vi "MT EbN0 Calculation(ASK).vi"(0 "Recieved waveform":T3={"t0"=0.0, "dt"=1.0, "Y"=[]} {"Y" format="%.3f"; "dt" format="%^.2e"; "t0" format="%.4f"}, 1 "pulse shaping filter coefficients":dbl[](array[numeric]) format="%.2f", 5 "ASK system parameters":T1={"samples per symbol (16)"=16, "symbol map"=[]} {"symbol map" format="%.3f"}, 7 "synchronization parameters":T2 {"sync sequence" format="%.2f"}, 9 "matched filter coefficients":dbl[](array[numeric]) format="%.2f", 11 "error in (no error)":errorcluster, 12 "reset? (T)":bool=TRUE) -> (4 "Eb/N0":dbl, 6 "Eb/N0(dB)":dbl, 15 "error out":errorcluster)   [LabVIEW 2020, in "niDMT.lvlib"]
uses:
  <vilib>/addons/Modulation/niDMT.lvlib
  <vilib>/addons/Modulation/Analog/controls/Complex Data Waveform.ctl
  <vilib>/Analysis/2dsp.llb/1D Convolution (DBL).vi
  <vilib>/Analysis/NI_AALPro.lvlib
  <vilib>/addons/Modulation/niAMT.lvlib
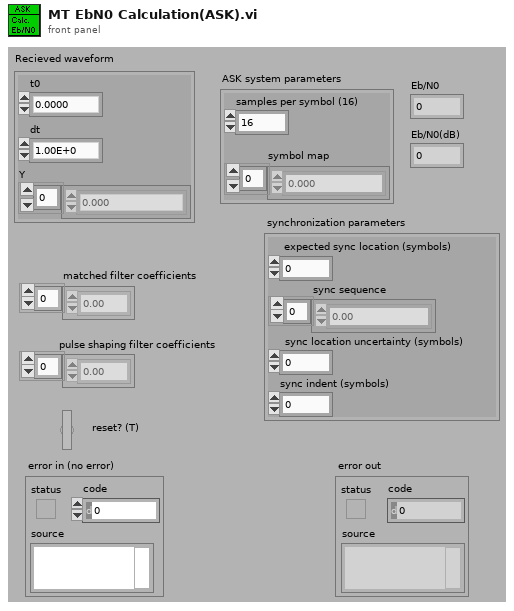
[diagram p1: front panel]
types:
  T1 = cluster{"samples per symbol (16)":i32, "symbol map":cdb[]}
  T2 = cluster{"expected sync location (symbols)":i32, "sync sequence":cdb[], "sync location uncertainty (symbols)":i32, "sync indent (symbols)":i32}
  T3 = typedef "niAMT.lvlib/Complex Data Waveform.ctl" = cluster{"t0":dbl, "dt":dbl, "Y":cdb[]}
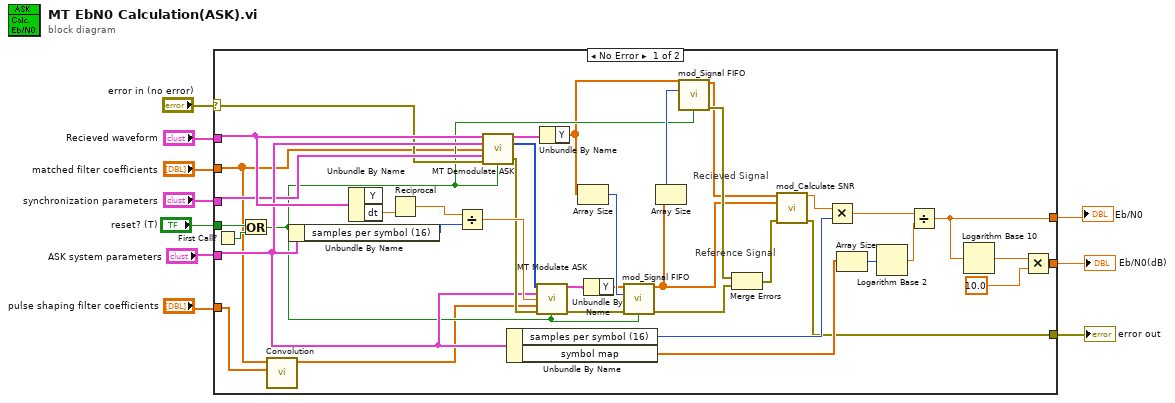
[diagram p0: block diagram]
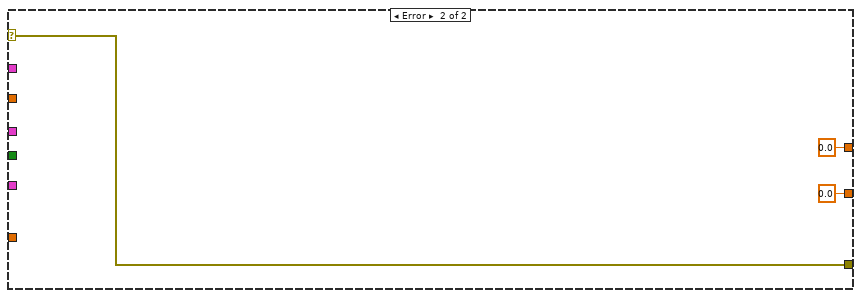
[diagram p2: hidden frame]
diagram:
  n1 = case shown="No Error" "error in (no error)" {
    selector: "error in (no error)" -> [w19 w52]
    tunnel: "matched filter coefficients" -> [w15 _]
    tunnel: "pulse shaping filter coefficients" -> [w14 _]
    tunnel: [w35 0.0] -> w8
    tunnel: [w32 0.0] -> w7
    tunnel: "Recieved waveform" -> [w27 _]
    tunnel: "ASK system parameters" -> [w26 _]
    tunnel: "synchronization parameters" -> [w25 _]
    tunnel: [w20 w52] -> w3
    tunnel: "reset? (T)" -> [w18 _]
    frame No Error {
      # "Recieved Signal"
      # "Reference Signal"
      n2 = First Call?() -> (First Call?: T/F=w17:bool)
      n3 = Or(x=w18, y=w17) -> (x .or. y?=w16:bool)
      n4 = call-poly <vilib>:"Convolution.vi"("Y"=w14, "X"=w15) -> ("X * Y"=w13:dbl[])  [unwired: 1 in, 8 out]
      n5 = Unbundle By Name(w26) -> ("samples per symbol (16)"=w47:i32)
      n6 = Unbundle By Name(w27) -> ("dt"=w49:dbl)  [unwired: 1 out]
      n7 = Reciprocal(x=w49) -> (1/x=w45:dbl)
      n8 = Divide(x=w45, y=w47) -> (x/y=w48:dbl)
      n9 = call <vilib>:"MT Demodulate ASK.vi"("input complex waveform"=w27, "ASK system parameters"=w26, "matched filter coefficients"=w15, "synchronization parameters"=w25, "error in (no error)"=w19, "reset? (T)"=w16) -> ("recovered complex waveform"=w12:T3, "output bit stream"=w42:i8[], "error out"=w31:errorcluster)  [unwired: 1 in, 6 out]
      n10 = Unbundle By Name(w26) -> ("samples per symbol (16)"=w46:i32, "symbol map"=w44:cdb[])
      n11 = call <vilib>:"MT Modulate ASK.vi"("input bit stream"=w42, "ASK system parameters"=w26, "symbol rate (Hz)"=w48, "pulse shaping filter coefficients"=w13, "error in (no error)"=w31, "reset? (T)"=w16) -> ("output complex waveform"=w40:T3, "error out"=w30:errorcluster)  [unwired: 1 in, 7 out]
      n12 = Unbundle By Name(w12) -> ("Y"=w11:cdb[])
      n13 = Array Size(array=w11) -> (size(s)=w39:i32)
      n14 = Unbundle By Name(w40) -> ("Y"=w38:cdb[])
      n15 = call <vilib>:"mod_Signal FIFO.vi"("Signal In"=w38, "Output Length"=w39, "error in (no error)"=w30, "Reset? (T)"=w16) -> ("Signal Out"=w23:cdb[], "error out"=w28:errorcluster)  [unwired: 10 out]
      n16 = Array Size(array=w23) -> (size(s)=w37:i32)
      n17 = call <vilib>:"mod_Signal FIFO.vi"("Signal In"=w11, "Output Length"=w37, "Reset? (T)"=w16) -> ("Signal Out"=w24:cdb[], "error out"=w29:errorcluster)  [unwired: 1 in, 10 out]
      n18 = Merge Errors(w29, w28) -> (w21:errorcluster)
      n19 = call <vilib>:"mod_Calculate SNR.vi"("Recieved Waveform"=w24, "Reference Waveform"=w23, "error in (no error)"=w21) -> ("SNR"=w22:dbl, "error out"=w20:errorcluster)  [unwired: 11 out]
      n20 = Multiply(x=w22, y=w46) -> (x*y=w41:dbl)
      n21 = Array Size(array=w44) -> (size(s)=w43:i32)
      n22 = Logarithm Base 2(1:w43) -> (0:w36:dbl)
      n23 = Divide(x=w41, y=w36) -> (x/y=w35:dbl)
      n24 = Logarithm Base 10(1:w35) -> (0:w34:dbl)
      n25 = Multiply(x=w34, y=10.0) -> (x*y=w32:dbl)
    }
    frame Error {
    }
  }
  "Eb/N0" <- w8
  "Eb/N0(dB)" <- w7
  "error out" <- w3
